vi "Database-GetDBstatus.vi"(1 "Idx":i32) -> (0 "Status":T1)   [LabVIEW 2016]
uses:
  Database.Global.vi
  Database.Data.Status.ctl
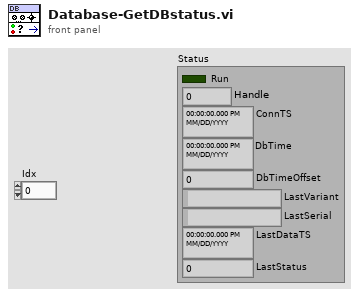
[diagram p1: front panel]
types:
  T1 = typedef "Database.Data.Status.ctl" = cluster{"Run":bool, "Handle":i32, "ConnTS":timestamp, "DbTime":timestamp, "DbTimeOffset":dbl, "LastVariant":string, "LastSerial":string, "LastDataTS":timestamp, "LastStatus":i32}
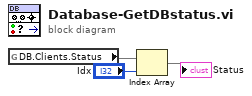
[diagram p0: block diagram]
diagram:
  n1 = global read "Database.Global.vi" "DB.Clients.Status"() -> (w3)
  n2 = Index Array(array=w3, index="Idx") -> (element=→"Status")
